vi "MainStateMachine.vi"(8 "error constant":errorcluster, 11 "FPGA VI Reference In":refnum<k20>) -> (0 "error constant 2":errorcluster, 3 "FPGA VI Reference Out":refnum<k20>)   [LabVIEW 2018]
uses:
  Type_Def/Type_Def ControlState.ctl
  Type_Def/Type_Def Actuator Controls.ctl
  Type_Def/Type_Def Master_DataControl.ctl
  Type_Def/TypeDef_cRIOData.ctl
  Type_Def/Type_Def IMUData.ctl
  Type_Def/TypeDef_BMSData.ctl
  Type_Def/TypeDef_BmsStatus.ctl
  Type_Def/TypeDef FixedMotorData.ctl
  <vilib>/Platform/TimedLoop/XDataNode/timing_clust.ctl
  <vilib>/Platform/TimedLoop/XDataNode/nitl_modes.ctl
  <vilib>/Platform/TimedLoop/XDataNode/wakeup.ctl
  <vilib>/Platform/TimedLoop/XDataNode/loadnilvce.vi
  <vilib>/platform/TimedLoop/XDataNode/XDataNode.xnode
  <vilib>/Platform/TimedLoop/XDataNode/XDNodeRunTimeDep.lvlib
panel:
  in  "Velocity":dbl
  in  "Displacement":dbl
  in  "Launch":bool
  in  "ForceIdle":bool
  out "Current State":T1
  in  "stop":bool
  in  "Shutdown":bool
  in  "Vent":bool
  in  "Service":bool
  in  "Ready":bool
  in  "SystemCheck":bool
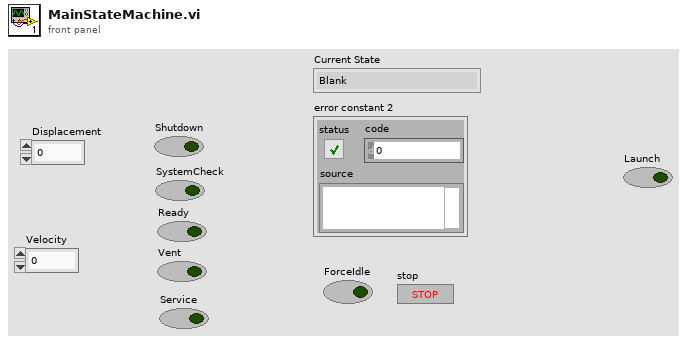
[diagram p1: front panel]
types:
  T1 = typedef "Type_Def ControlState.ctl" = enum16{"Blank", "Systems Check", "Idle", "Ready", "Pushing", "CrawlingPrecharge", "Braking", "Fault", "Boot Up", "Unpowered", "Crawling", "Shutdown", "Service Push", "Service Wait", "Vent", "Precharge"}
  T2 = typedef "Type_Def Actuator Controls.ctl" = cluster{"Reverse ":bool, "Precharge Ctrl":bool, "Pump Ctrl":bool, "24 VDC Ctr":bool, "Vent Solenoid":bool, "Brake Solenoid":bool, "EMCY  Brake Solenoid":bool, "Digital Out 7B ":bool, "Forward Ctrl":bool, "Contact H1":bool, "Contact L1":bool, "Contact H2":bool, "Contact L2 ":bool, "LED RED":bool, "LED GREEN":bool, " Digital Out 7A":bool}
  T3 = typedef "Type_Def Master_DataControl.ctl" = cluster{"cRIO Data":T4, "IMU Data":T5, "BMS Data":T6, "Motor Data":T8}
  T4 = typedef "TypeDef_cRIOData.ctl" = cluster{"HallEffect Right (cm)":dbl, "HallEffect Left (cm)":dbl, "Optical Sensor 1 (V)":dbl, "Optical Sensor 2 (V)":dbl, "24V Battery (V)":dbl, "24V Current (A)":dbl, "Contactor H1 Continuity":dbl, "Contactor L1 Continuity ":dbl, "Contactor H2 Continuity":dbl, "Contactor L2 Continuity ":dbl, "Time (ms)":dbl, "Displacement (ft)":dbl, "Velocity (ft/s)":dbl, "ABS Pressure 1 (psig)":dbl, "ABS Pressure 2 (psig) ":dbl, "24 Temp Thermistor 1 (C)":dbl, "24 Temp Thermistor 2 (C) ":dbl, "24 Temp Thermistor  3 (C) ":dbl, "24 Temp Thermistor 4 (C) ":dbl, "Brake PT(psig)":dbl, "Tank PT(psig) ":dbl, "Pump PT(psig)":dbl, "24 Temp Average(C) ":dbl, "High Voltage 1":bool}
  T5 = typedef "Type_Def IMUData.ctl" = cluster{"x acceleration (g)":dbl, "Pressure (psia)":dbl, "Temperature (F)":dbl}
  T6 = typedef "TypeDef_BMSData.ctl" = cluster{"Max Cell Voltage (V)":dbl, "Max Cell ID":dbl, "Min Cell Voltage (V)":dbl, "Min Cell ID":dbl, "State of Charge (%)":dbl, "Average Voltage (V)":dbl, "Voltage Delta (V)":dbl, "Pack Current (A)":dbl, "Pack Voltage (V)":dbl, "Max Resistance (Ohm)":dbl, "Min Resistance (Ohm)":dbl, "Average Resistance (Ohm)":dbl, "Delta Resistance (Ohm)":dbl, "Highest Temperature(F)":dbl, "BmsStatus":T7}
  T7 = typedef "TypeDef_BmsStatus.ctl" = cluster{"isFault":bool, "isolationMonitoring":bool}
  T8 = typedef "TypeDef FixedMotorData.ctl" = cluster{" Velocity (RPM)":dbl, " MotorTemp(C)":dbl, " ControlTemp(C)":dbl, " DcLinkVolt(V)":dbl, " ErrorCode":dbl, "IsAlive":bool, "motorStatus":cluster{"isReady":bool, "isOn":bool, "isOperEn":bool, "isFault":bool, "isVoltEn":bool, "targetReached":bool, "isWarning":bool}, "motorControllerState":u16}
  T9 = typedef "Type_Def ClusterSensor.ctl" = cluster{"Sensor Data":dbl, "Max":dbl, "Min":dbl, "Previous Data":dbl, "#same":dbl}
  T10 = typedef "XDNodeRunTimeDep.lvlib/timing_clust.ctl" = cluster{"Expected End [f-1]":u64, "Actual End [f-1]":u64, "Finished Late? [f-1]":bool, "Expected End [i-1]":u64, "Actual End [i-1]":u64, "Finished Late? [i-1]":bool, "Expected Start [i]":u64, "Actual Start [i]":u64, "Expected Start [f]":u64, "Actual Start [f]":u64, "Source Name":string, "Structure Name":string, "Period":i64, "Deadline":i64, "Offset":i64, "Start":i64, "Priority":i32, "Timeout":i32, "Mode":T11, "Wakeup Reason":T12, "Error":errorcluster, "Source Type":string, "Secondary Source Type":string, "Global End Time":u64, "Global Start Time":u64, "Frame Duration":u64, "Iteration Duration":u64, "Assigned CPU":i32, "I/O Scan Engine Mode":u32}
  T11 = typedef "XDNodeRunTimeDep.lvlib/nitl_modes.ctl" = enum32{"No Change", "Process missed periods, maintain original phase", "Discard missed periods, maintain original phase", "Process missed periods, ignore original phase", "Discard missed periods, ignore original phase"}
  T12 = typedef "XDNodeRunTimeDep.lvlib/wakeup.ctl" = enum32{"Normal", "Aborted", "Asynchronous wakeup", "Timing source error", "Timed loop error", "Timeout"}
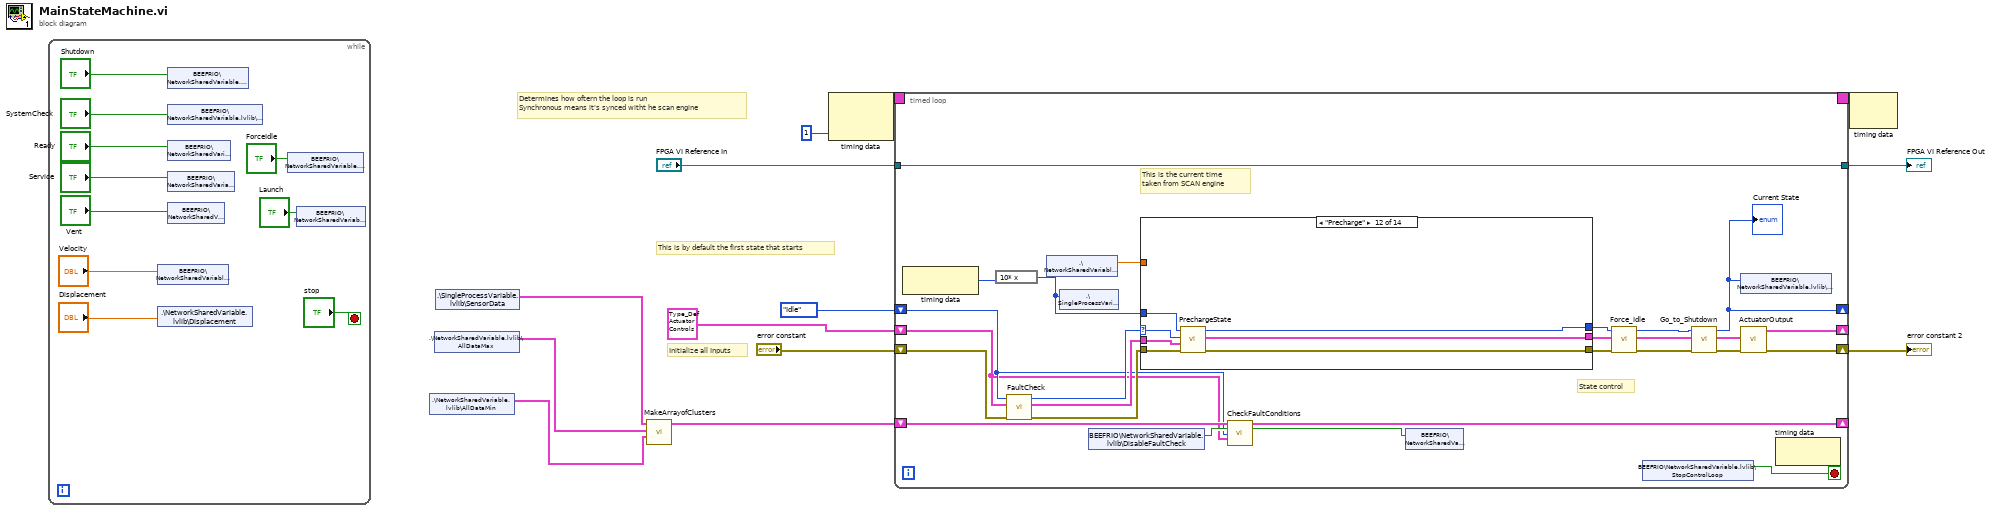
[diagram p0: block diagram]
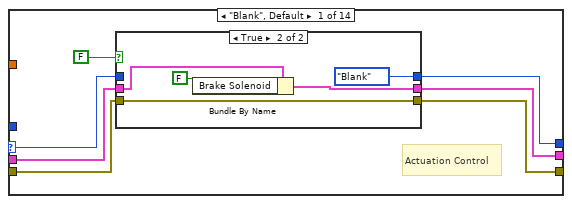
[diagram p2: hidden frame]
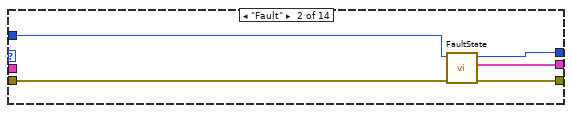
[diagram p4: hidden frame]
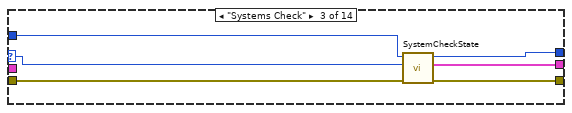
[diagram p5: hidden frame]
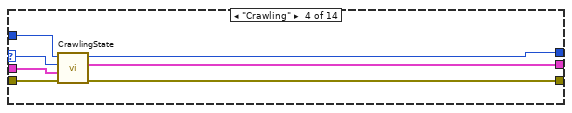
[diagram p6: hidden frame]
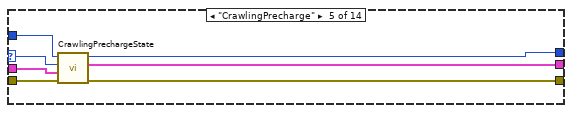
[diagram p7: hidden frame]
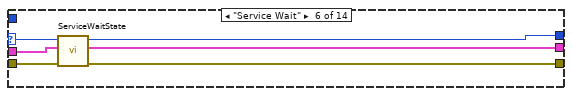
[diagram p8: hidden frame]
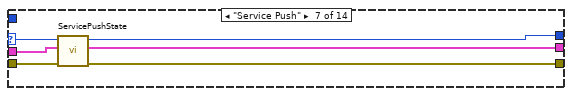
[diagram p9: hidden frame]
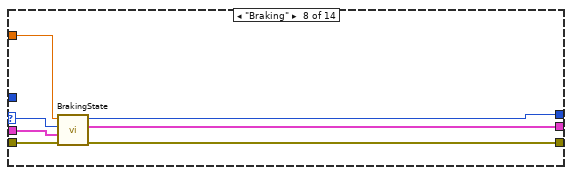
[diagram p10: hidden frame]
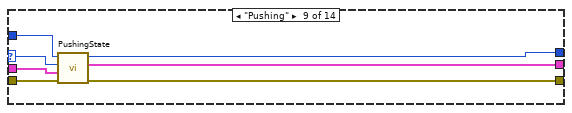
[diagram p11: hidden frame]
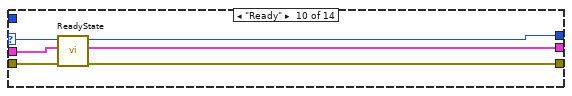
[diagram p12: hidden frame]
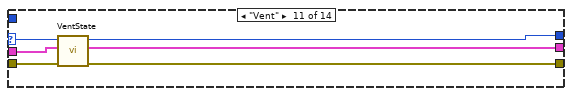
[diagram p13: hidden frame]
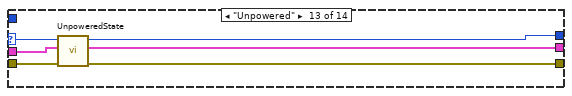
[diagram p14: hidden frame]
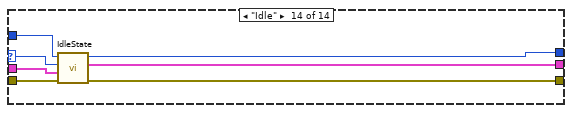
[diagram p15: hidden frame]
diagram:
  # "Determines how oftern the loop is run \nSynchronous means it's synced witht he scan engine"
  # "Initialize all Inputs"
  # "This is by default the first state that starts"
  n1 = while {
    stop <- "stop" stop-if-true
    n2 = shared-variable "BEEFRIO\\NetworkSharedVariable.lvlib\\Velocity"("Velocity") -> ()  [unwired: 1 in, 1 out]
    n3 = shared-variable ".\\NetworkSharedVariable.lvlib\\Displacement"("Displacement") -> ()  [unwired: 1 in, 1 out]
    n4 = shared-variable "BEEFRIO\\NetworkSharedVariable.lvlib\\Shutdown"("Shutdown") -> ()  [unwired: 1 in, 1 out]
    n5 = shared-variable "BEEFRIO\\NetworkSharedVariable.lvlib\\SystemCheck"("SystemCheck") -> ()  [unwired: 1 in, 1 out]
    n6 = shared-variable "BEEFRIO\\NetworkSharedVariable.lvlib\\Ready"("Ready") -> ()  [unwired: 1 in, 1 out]
    n7 = shared-variable "BEEFRIO\\NetworkSharedVariable.lvlib\\Service"("Service") -> ()  [unwired: 1 in, 1 out]
    n8 = shared-variable "BEEFRIO\\NetworkSharedVariable.lvlib\\Vent"("Vent") -> ()  [unwired: 1 in, 1 out]
    n9 = shared-variable "BEEFRIO\\NetworkSharedVariable.lvlib\\ForceIdle"("ForceIdle") -> ()  [unwired: 1 in, 1 out]
    n10 = shared-variable "BEEFRIO\\NetworkSharedVariable.lvlib\\Launch"("Launch") -> ()  [unwired: 1 in, 1 out]
  }
  n11 = shared-variable ".\\NetworkSharedVariable.lvlib\\AllDataMin"() -> (w2:T3)  [unwired: 1 in, 1 out]
  n12 = shared-variable ".\\NetworkSharedVariable.lvlib\\AllDataMax"() -> (w3:T3)  [unwired: 1 in, 1 out]
  n13 = shared-variable ".\\SingleProcessVariable.lvlib\\SensorData"() -> (w1:T3)  [unwired: 1 in, 1 out]
  n14 = call "MakeArrayofClusters.vi"("AllDataMin"=w2, "AllDataMax"=w3, "SensorData"=w1) -> ("Array"=w8:cluster{"SensorCluster":T9}[])  [unwired: 8 in]
  n15 = node-c288 ("Input Node")(i64 1 ("Period")) -> (w13:T10)  [unwired: 1 in]
  n16 = timed-loop "Timed Loop" {
    timing: w13 -> [_]
    timing-out: [_] -> w12
    shift-right: [w26] -> _
    shift-left: Type_Def_ControlState."Idle" -> [w34]
    shift-right: [w43] -> _
    shift-left: T2 {"Reverse "=FALSE, "Precharge Ctrl"=FALSE, "Pump Ctrl"=FALSE, "24 VDC Ctr"=FALSE, "Vent Solenoid"=FALSE, "Brake Solenoid"=FALSE, "EMCY  Brake Solenoid"=FALSE, "Digital Out 7B "=FALSE, "Forward Ctrl"=FALSE, "Contact H1"=FALSE, "Contact L1"=FALSE, "Contact H2"=FALSE, "Contact L2 "=FALSE, "LED RED"=FALSE, "LED GREEN"=FALSE, " Digital Out 7A"=FALSE} -> [w32]
    shift-right: [w42] -> w5
    shift-left: "error constant" -> [w49]
    shift-right: [w37] -> _
    shift-left: w8 -> [w36]
    tunnel: [w30] -> w7
    tunnel: "FPGA VI Reference In" -> [w30]
    stop <- w31 stop-if-true
    # "State control"
    # "This is the current time \ntaken from SCAN engine"
    n17 = node-c288() -> (w45:i64)  [unwired: 1 in]
    n18 = expression code="10* x"(w45) -> (w44:i64)
    n19 = call "FaultCheck.vi"("error in (no error)"=w49, "Cluster in"=w32, "Enum in"=w34) -> ("error out"=w38:errorcluster, "Cluster out"=w39:T2, "Enum out"=w40:T1)  [unwired: 6 in]
    n20 = shared-variable ".\\NetworkSharedVariable.lvlib\\Velocity"() -> (w41:dbl)  [unwired: 1 in, 1 out]
    n21 = shared-variable ".\\SingleProcessVariable.lvlib\\Time"(w44) -> ()  [unwired: 1 in, 1 out]
    n22 = shared-variable "BEEFRIO\\NetworkSharedVariable.lvlib\\DisableFaultCheck"() -> (w35:bool)  [unwired: 1 in, 1 out]
    n23 = case shown="\"Precharge\"" w40 {
      selector: w40 -> [w56 _ w70 w82 w89 w95 w101 w108 w115 w121 w127 w134 w140 w147]
      tunnel: [w55 w67 w73 w81 w88 w94 w100 w107 w114 w120 w126 w133 w139 w146] -> w46
      tunnel: [w53 w65 w71 w79 w86 w92 w98 w105 w112 w118 w124 w131 w137 w144] -> w48
      tunnel: w39 -> [w54 _ _ w80 w87 w93 w99 w106 w113 w119 w125 w132 w138 w145]
      tunnel: [w52 w66 w72 w78 w85 w91 w97 w104 w111 w117 w123 w130 w136 w143] -> w47
      tunnel: w38 -> [w51 w69 w74 w77 w84 w90 w96 w103 w110 w116 w122 w129 w135 w142]
      tunnel: w44 -> [_ w68 w75 w76 w83 _ _ _ w109 _ _ w128 _ w141]
      tunnel: w41 -> [_ _ _ _ _ _ _ w102 _ _ _ _ _ _]
      frame "Blank", Default {
        # "Actuation Control"
        n24 = case shown="True" FALSE {
          tunnel: w56 -> [w59 _]
          tunnel: [w59 Type_Def_ControlState."Blank"] -> w55
          tunnel: w54 -> [w58 w63]
          tunnel: [w58 w61] -> w53
          tunnel: [w57 w60] -> w52
          tunnel: w51 -> [w57 w60]
          frame False {
          }
          frame True {
            n25 = Bundle By Name(cluster=w63, "Brake Solenoid"=FALSE ("Digital Out 5")) -> (w61:T2)
          }
        }
      }
      frame "Fault" {
        n26 = call "FaultState.vi"("error in (no error)"=w69, "Actual Start [i]"=w68) -> ("error out"=w66:errorcluster, "Cluster"=w65:T2, "Numeric"=w67:i64)  [unwired: 7 in]
      }
      frame "Systems Check" {
        n27 = call "SystemCheckState.vi"("error in (no error)"=w74, "State in"=w70, "Actual Start [i]"=w75) -> ("error out"=w72:errorcluster, "Cluster"=w71:T2, "State Out"=w73:T1)  [unwired: 5 in]
      }
      frame "Crawling" {
        n28 = call "CrawlingState.vi"("error in (no error)"=w77, "Cluster in"=w80, "Enum in"=w82, "Actual Start [i]"=w76) -> ("error out"=w78:errorcluster, "Cluster out"=w79:T2, "Enum"=w81:T1)  [unwired: 5 in]
      }
      frame "CrawlingPrecharge" {
        n29 = call "CrawlingPrechargeState.vi"("error in (no error)"=w84, "Cluster in"=w87, "Enum in"=w89, "Actual Start [i]"=w83) -> ("error out"=w85:errorcluster, "Cluster out"=w86:T2, "Enum"=w88:T1)  [unwired: 5 in]
      }
      frame "Service Wait" {
        n30 = call "ServiceWaitState.vi"("error in (no error)"=w90, "Cluster in"=w93, "Enum in"=w95) -> ("error out"=w91:errorcluster, "Cluster out"=w92:T2, "Enum"=w94:T1)  [unwired: 6 in]
      }
      frame "Service Push" {
        n31 = call "ServicePushState.vi"("error in (no error)"=w96, "Cluster in"=w99, "Enum in"=w101) -> ("error out"=w97:errorcluster, "Cluster out"=w98:T2, "Enum out"=w100:T1)  [unwired: 6 in]
      }
      frame "Braking" {
        n32 = call "BrakingState.vi"("error in (no error)"=w103, "Cluster in"=w106, "Enum in"=w108, "Velocity"=w102) -> ("error out"=w104:errorcluster, "Cluster"=w105:T2, "Enum"=w107:T1)  [unwired: 5 in]
      }
      frame "Pushing" {
        n33 = call "PushingState.vi"("error in (no error)"=w110, "Cluster in"=w113, "Enum in"=w115, "Actual Start [i]"=w109) -> ("error out"=w111:errorcluster, "Cluster out"=w112:T2, "Enum"=w114:T1)  [unwired: 5 in]
      }
      frame "Ready" {
        n34 = call "ReadyState.vi"("error in (no error)"=w116, "Cluster in"=w119, "Enum in"=w121) -> ("error out"=w117:errorcluster, "Cluster out"=w118:T2, "Enum"=w120:T1)  [unwired: 6 in]
      }
      frame "Vent" {
        n35 = call "VentState.vi"("error in (no error)"=w122, "Cluster in"=w125, "Enum in"=w127) -> ("error out"=w123:errorcluster, "Cluster out"=w124:T2, "Enum out"=w126:T1)  [unwired: 6 in]
      }
      frame "Precharge" {
        n36 = call "PrechargeState.vi"("error in (no error)"=w129, "Cluster in"=w132, "Enum in"=w134, "Actual Start [i]"=w128) -> ("error out"=w130:errorcluster, "Cluster out"=w131:T2, "Enum"=w133:T1)  [unwired: 5 in]
      }
      frame "Unpowered" {
        n37 = call "UnpoweredState.vi"("error in (no error)"=w135, "Cluster in"=w138, "Enum in"=w140) -> ("error out"=w136:errorcluster, "Cluster out"=w137:T2, "Enum"=w139:T1)  [unwired: 6 in]
      }
      frame "Idle" {
        n38 = call "IdleState.vi"("error in (no error)"=w142, "Cluster in"=w145, "Enum in"=w147, "Actual Start [i]"=w141) -> ("error out"=w143:errorcluster, "Cluster out"=w144:T2, "Enum"=w146:T1)  [unwired: 5 in]
      }
    }
    n39 = call "CheckFaultConditions.vi"("Array 2"=w36, "DisableFaultCheck"=w35, "ControlState"=w34, 9:w32) -> ("Array out"=w37:cluster{"SensorCluster":T9}[], "Fault?"=w33:bool)  [unwired: 10 in]
    n40 = shared-variable "BEEFRIO\\NetworkSharedVariable.lvlib\\Fault"(w33) -> ()  [unwired: 1 in, 1 out]
    n41 = call "Force_Idle.vi"("error in (no error)"=w47, "Cluster in"=w48, "Enum in"=w46) -> ("error out"=w25:errorcluster, "Cluster out"=w29:T2, "Enum out"=w27:T1)  [unwired: 6 in]
    n42 = shared-variable "BEEFRIO\\NetworkSharedVariable.lvlib\\StopControlLoop"() -> (w31:bool)  [unwired: 1 in, 1 out]
    n43 = call "Go_to_Shutdown.vi"("error in (no error)"=w25, "Cluster in"=w29, "Enum in"=w27) -> ("error out"=w24:errorcluster, "Cluster out"=w28:T2, "Enum out"=w26:T1)  [unwired: 5 in, 1 out]
    "Current State" <- w26
    n44 = shared-variable "BEEFRIO\\NetworkSharedVariable.lvlib\\CurrentState"(w26) -> ()  [unwired: 1 in, 1 out]
    n45 = call "ActuatorOutput.vi"("error in (no error)"=w24, "Cluster in"=w28) -> ("error out"=w42:errorcluster, "Cluster"=w43:T2)  [unwired: 8 in]
    n46 = node-c288() -> ()  [unwired: 1 in, 1 out]
  }
  "FPGA VI Reference Out" <- w7
  "error constant 2" <- w5
  n47 = node-c288(w12) -> ()  [unwired: 1 out]
